vi "SPI Close.vi"(8 "Error In":errorcluster, 11 "SPI Configuration In":T1={"CLK Frequency (Hz)"=250000, "CPOL"=FALSE, "CPHA"=FALSE, "CS Channel"="", "CLK Channel"="", "MOSI Channel"="", "MISO Channel"="", "Active CS"=FALSE, "Dig In Task"="", "Dig Out Task"=""} {"CLK Frequency (Hz)" format="%#.6p"}) -> (0 "Error Out":errorcluster, 3 "SPI Configuration Out":T1={"CLK Frequency (Hz)"=250000, "CPOL"=FALSE, "CPHA"=FALSE, "CS Channel"="", "CLK Channel"="", "MOSI Channel"="", "MISO Channel"="", "Active CS"=FALSE, "Dig In Task"="", "Dig Out Task"=""} {"CLK Frequency (Hz)" format="%#.6p"})   [LabVIEW 2016, in "SPIVI.lvlib"]
uses:
  SPIVI.lvlib
  Typedefs/SPI Configuration.ctl
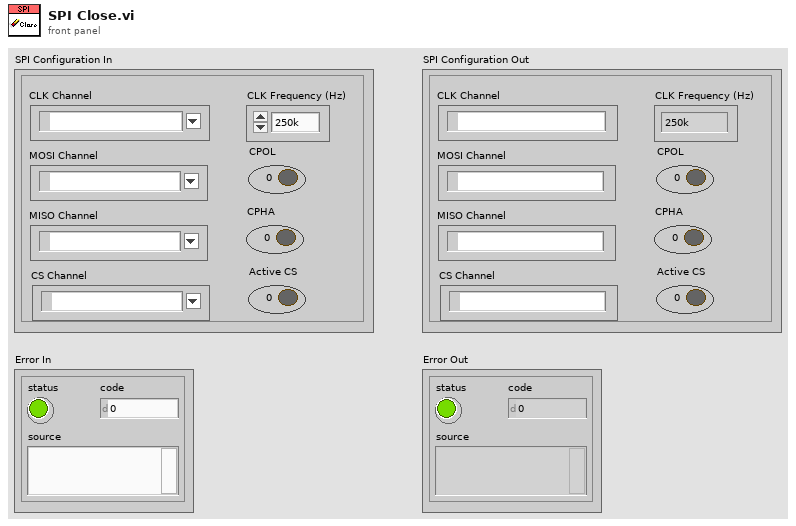
[diagram p1: front panel]
types:
  T1 = typedef "SPIVI.lvlib/SPI Configuration.ctl" = cluster{"CLK Frequency (Hz)":u32, "CPOL":bool, "CPHA":bool, "CS Channel":tag, "CLK Channel":tag, "MOSI Channel":tag, "MISO Channel":tag, "Active CS":bool, "Dig In Task":refnum<k21>, "Dig Out Task":refnum<k21>}
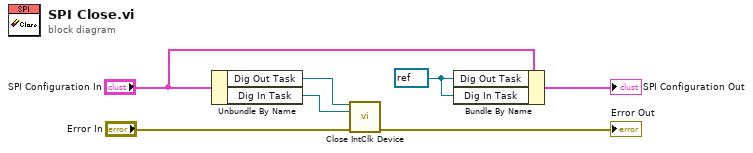
[diagram p0: block diagram]
diagram:
  w3 = refnum<k21> refnum ("Dig Out Task")
  n1 = Unbundle By Name("SPI Configuration In") -> ("Dig Out Task"=w5:refnum<k21>, "Dig In Task"=w4:refnum<k21>)
  n2 = call "Close IntClk Device.vi"("Dig out task"=w5, "Dig in task"=w4, "error in"="Error In") -> ("error out"=→"Error Out":errorcluster)  [unwired: 12 in]
  n3 = Bundle By Name(cluster="SPI Configuration In", "Dig Out Task"=w3, "Dig In Task"=w3) -> (→"SPI Configuration Out":T1)
